vi "Config LogicIO.vi"(8 "error in (no error)":errorcluster, 11 "Configuration in":refnum<class "Configuration.lvclass">) -> (0 "error out":errorcluster, 3 "Configuration out":refnum<class "Configuration.lvclass">)   [LabVIEW 2016, in "Hardware.lvlib" / "LogicIO.lvlib" / "LogicIO Configuration.lvclass"]
uses:
  <userlib>/Common Components/Hardware/LogicIO/LogicIO Config/LogicIO Configuration.lvclass
  <userlib>/Configuration Dialog Actor/Configuration.lvclass
  C:/Program Files (x86)/National Instruments/LabVIEW 2016/user.lib/Configuration Dialog Actor/Configuration.lvclass
  <userlib>/Common Components/Hardware/LogicIO/LogicIO Config/LogicIO Configuration.lvclass/LogicIO Configuration.ctl
  <userlib>/Common Components/Hardware/Abstract Hardware/Hardware.lvclass/Hardware.ctl
  <userlib>/Common Components/Hardware/DevInfo/DevInfo.lvclass/DevInfo.ctl
  <userlib>/Common Components/Hardware/Abstract Hardware/Read DevInfo.vi
  <userlib>/Common Components/Hardware/DevInfo/Read COMM Address.vi
  <userlib>/Common Components/Hardware/DevInfo/Read Sub-COMM Address.vi
  <userlib>/Common Components/Hardware/DevInfo/Read HW Type.vi
  <userlib>/Common Components/Hardware/DevInfo/Read Device Name.vi
  <userlib>/Common Components/Hardware/LogicIO/LogicIO/LogicIO.lvclass
  C:/Program Files (x86)/National Instruments/LabVIEW 2016/user.lib/Common Components/Hardware/Abstract Hardware/Hardware.lvclass
  <userlib>/Common Components/Hardware/DevInfo/DevInfo.lvclass
panel:
  out "Status":bool
  out "HW Type":string
  out "Sub-COMM Address":string
  out "COMM Address":string
  out "Device Name":string
  in  "Revert":bool
  in  "Apply":bool
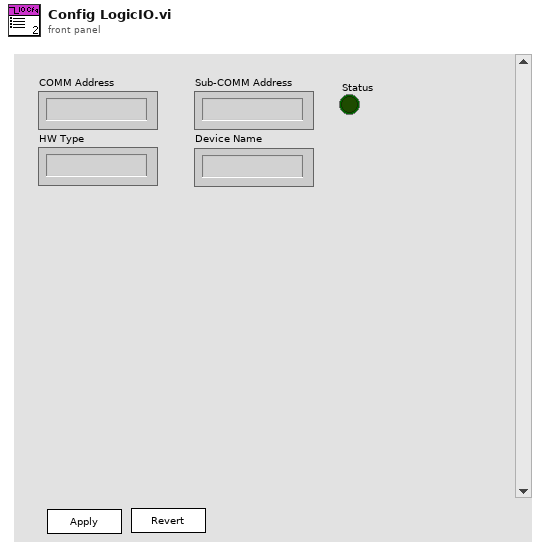
[diagram p1: front panel]
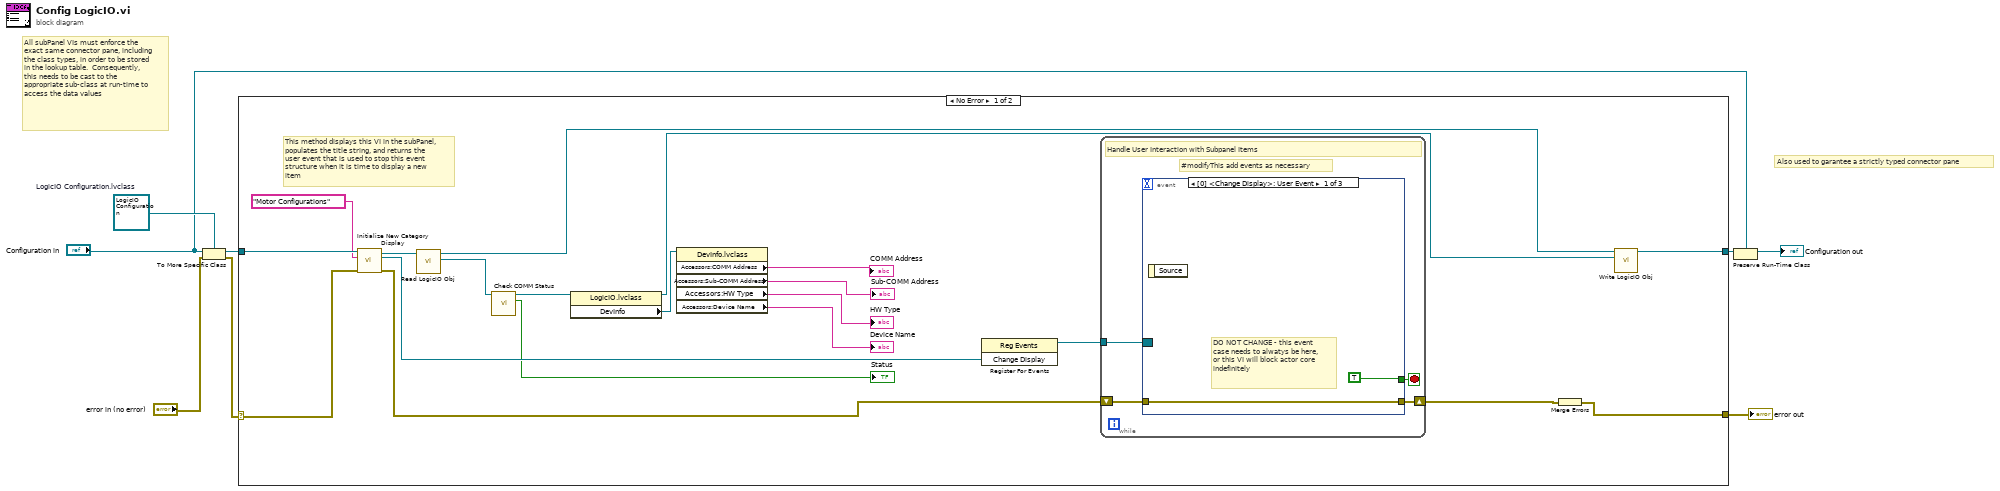
[diagram p0: block diagram]
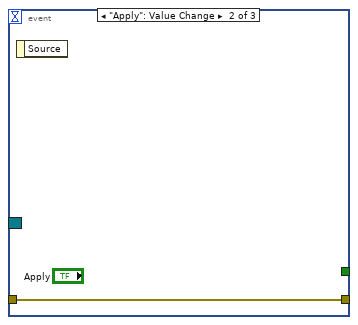
[diagram p2: hidden frame]
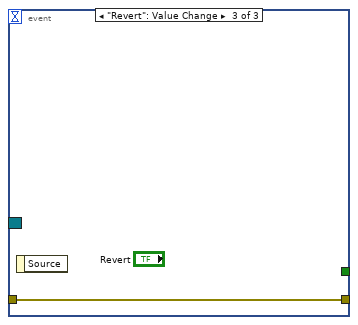
[diagram p3: hidden frame]
diagram:
  w5 = refnum<class "LogicIO Configuration.lvclass"> refnum  # LogicIO Configuration.lvclass
  # "Also used to garantee a strictly typed connector pane"
  # "All subPanel VIs must enforce the exact same connector pane, including the class types, in order to be stored in the lookup table.  Consequently, this needs to be cast to the appropriate sub-class at run-time to access the data values"
  n1 = To More Specific Class(target class=w5, reference="Configuration in", error in="error in (no error)") -> (specific class reference=w6:refnum<class "LogicIO Configuration.lvclass">, error out=w1:errorcluster)
  n2 = case shown="No Error" w1 {
    selector: w1 -> [w23 w37]
    tunnel: w6 -> [w28 w38]
    tunnel: [w13 w38] -> w8
    tunnel: [w25 w37] -> w7
    frame No Error {
      # "This method displays this VI in the subPanel, populates the title string, and returns the user event that is used to stop this event structure when it is time to display a new item"
      n3 = call <userlib>:"Initialize New Category Display.vi"("error in (no error)"=w23, "Name to Display"="Motor Configurations", "Configuration in"=w28) -> ("error out"=w26:errorcluster, "Change Display"=w22:refnum<user-event>, "Configuration Out"=w27:refnum<class "LogicIO Configuration.lvclass">)  [unwired: 6 in]
      n4 = call <userlib>:"Read LogicIO Obj.vi"("LogicIO Configuration in"=w27) -> ("Hardware.lvlib:LogicIO.lvlib:LogicIO.lvclass"=w17:refnum<class "LogicIO.lvclass">, "LogicIO Configuration out"=w12:refnum<class "LogicIO Configuration.lvclass">)  [unwired: 9 in]
      n5 = call-dynamic "Check COMM Status.vi"("Hardware in"=w17) -> ("COMM status"=→"Status":bool, "Hardware out"=w11:refnum<class "LogicIO.lvclass">)  [unwired: 8 in, 1 out]
      n6 = property class="LogicIO.lvclass"(reference=w11) -> (reference out=w9:refnum<class "LogicIO.lvclass">, "DevInfo"=w16:refnum<class "DevInfo.lvclass">)  [unwired: 1 in, 1 out]
      n7 = property class="DevInfo.lvclass"(reference=w16) -> ("Accessors:COMM Address"=→"COMM Address":string, "Accessors:Sub-COMM Address"=→"Sub-COMM Address":string, "Accessors:HW Type"=→"HW Type":string, "Accessors:Device Name"=→"Device Name":string)  [unwired: 1 in, 2 out]
      n8 = register-events(w22) -> (reference out=w15:refnum<event-registration>)  [unwired: 2 in, 1 out]
      n9 = while {
        tunnel: w15 -> [w31]
        shift-right: [w30] -> w14
        shift-left: w26 -> [w29]
        stop <- w32 stop-if-true
        # "#modifyThis add events as necessary"
        # "Handle User Interaction with Subpanel Items"
        n10 = event shown="[0] <Change Display>: User Event" {
          selector: w31 -> [_ _ _]
          dyn-events: _ -> [_ _ _]
          timeout: _ -> [_ _ _]
          tunnel: [TRUE _ _] -> w32
          tunnel: [w33 w35 w36] -> w30
          tunnel: w29 -> [w33 w35 w36]
          event User Event {
            # "DO NOT CHANGE - this event case needs to alwatys be here, or this VI will block actor core indefinitely"
            n11 = event-data() -> ()  [unwired: 1 in, 1 out]
          }
          event "Apply": Value Change {
            n12 = event-data() -> ()  [unwired: 1 in, 1 out]
          }
          event "Revert": Value Change {
            n13 = event-data() -> ()  [unwired: 1 in, 1 out]
          }
        }
      }
      n14 = Merge Errors(w14) -> (w25:errorcluster)
      n15 = call <userlib>:"Write LogicIO Obj.vi"("Hardware.lvlib:LogicIO.lvlib:LogicIO.lvclass"=w9, "LogicIO Configuration in"=w12) -> ("LogicIO Configuration out"=w13:refnum<class "LogicIO Configuration.lvclass">)  [unwired: 9 in]
    }
    frame Error {
    }
  }
  "error out" <- w7
  n16 = Preserve Run-Time Class(object in=w8, 2:"Configuration in") -> (object out=→"Configuration out":refnum<class "Configuration.lvclass">)  [unwired: 1 in, 1 out]
